vi "PCO_GetSegmentImageSettings.vi"(0 "ph":u64, 5 "wSegment":u16, 11 "error in (no error)":errorcluster {"code" format="%x"}) -> (1 "wRoiX1":u16, 2 "wRoiX0":u16, 3 "wBinHorz":u16, 4 "ph out":u64, 6 "ErrorMessage":i32 format="%x", 8 "wXRes":u16, 10 "wYRes":u16, 12 "wRoiY1":u16, 13 "wRoiY0":u16, 14 "wBinVert":u16, 15 "error out":errorcluster {"code" format="%x"})   [LabVIEW 2020, in "SDK.lvlib" / "ImageInformation.lvlib"]
doc: "<b>Description:</b>\nInformation about previously recorded images is queried from the camera. The returned parameters depend on the camera settings which have been active during the last recording to the dedicated segment.\n\n<b>Supported camera type:</b>\npco.dimax, pco.1200, pco1600, pco.2000, pco.4000\n\n<b>Descriptor dependency:</b>\ndwGeneralCapsDESC1: NO_RECORDER"
uses:
  ImageInformation.lvlib
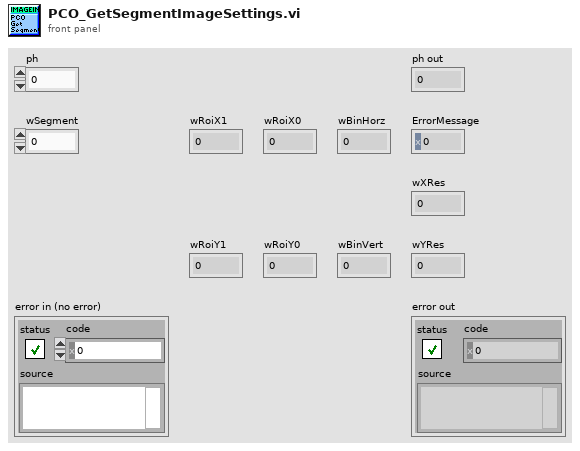
[diagram p1: front panel]
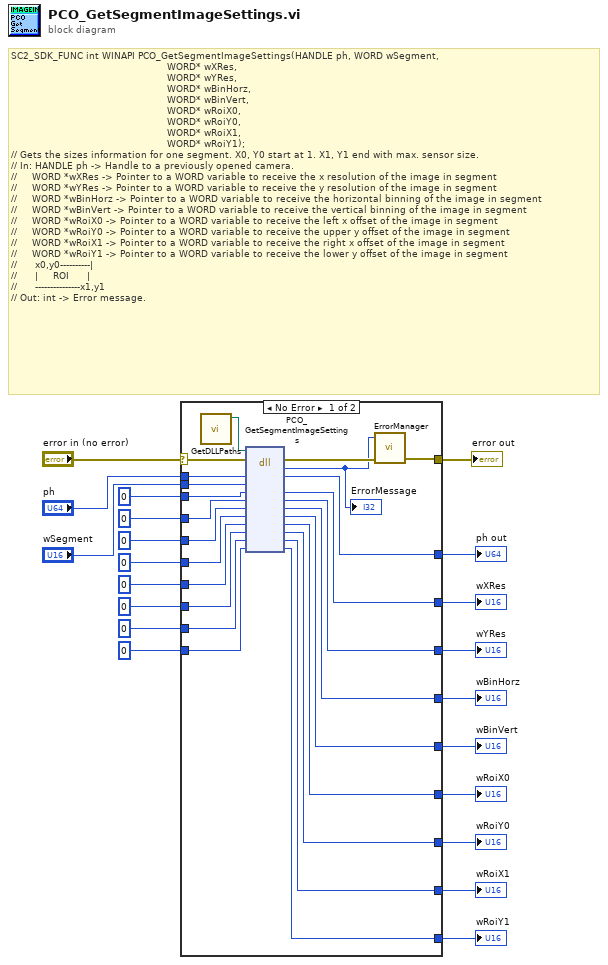
[diagram p0: block diagram]
diagram:
  # "SC2_SDK_FUNC int WINAPI PCO_GetSegmentImageSettings(HANDLE ph, WORD wSegment,\n                                                    WORD* wXRes,\n                                                    WORD* wYRes,\n                                                    WORD* wBinHorz,\n                                                    WORD* wBinVert,\n                                                    WORD* wRoiX0,\n                                                    WORD* wRoiY0,\n                                                    WORD* wRoiX1,\n                                                    WORD* wRoiY1);\n// Gets the sizes information for one segment. X0, Y0 start at 1. X1, Y1 end with max. sensor size.\n// In: HANDLE ph -> Handle to a previously opened camera.\n//     WORD *wXRes -> Pointer to a WORD variable to receive the x resolution of the image in segment\n//     WORD *wYRes -> Pointer to a WORD variable to receive the y resolution of the image in segment\n//     WORD *wBinHorz -> Pointer to a WORD variable to receive the horizontal binning of the image in segment\n//     WORD *wBinVert -> Pointer to a WORD variable to receive the vertical binning of the image in segment\n//     WORD *wRoiX0 -> Pointer to a WORD variable to receive the left x offset of the image in segment\n//     WORD *wRoiY0 -> Pointer to a WORD variable to receive the upper y offset of the image in segment\n//     WORD *wRoiX1 -> Pointer to a WORD variable to receive the right x offset of the image in segment\n//     WORD *wRoiY1 -> Pointer to a WORD variable to receive the lower y offset of the image in segment\n//      x0,y0----------|\n//      |     ROI      |\n//      ---------------x1,y1\n// Out: int -> Error message."
  n1 = case shown="No Error" "error in (no error)" {
    selector: "error in (no error)" -> [w23 w54]
    tunnel: "ph" -> [w45 w55]
    tunnel: [w44 w55] -> w20
    tunnel: "wSegment" -> [w43 _]
    tunnel: u16 0 ("wXRes") -> [w42 w53]
    tunnel: [w41 w53] -> w17
    tunnel: u16 0 ("wYRes") -> [w40 w52]
    tunnel: [w39 w52] -> w15
    tunnel: u16 0 ("wBinHorz") -> [w38 w51]
    tunnel: [w37 w51] -> w13
    tunnel: u16 0 ("wBinVert") -> [w36 w50]
    tunnel: [w35 w50] -> w11
    tunnel: u16 0 ("wRoiX0") -> [w34 w49]
    tunnel: [w33 w49] -> w9
    tunnel: u16 0 ("wRoiY0") -> [w32 w48]
    tunnel: [w31 w48] -> w7
    tunnel: u16 0 ("wRoiX1") -> [w30 w47]
    tunnel: [w29 w47] -> w5
    tunnel: u16 0 ("wRoiY1") -> [w28 w46]
    tunnel: [w27 w46] -> w3
    tunnel: [w25 w54] -> w2
    frame No Error {
      n2 = call "GetDLLPaths.vi"() -> ("SC2_Cam_Path"=w22:path)  [unwired: 9 in, 2 out]
      n3 = dll-call lib="?" fn="PCO_GetSegmentImageSettings"(path in=w22, error in=w23, "ph"=w45, "wSegment"=w43, "wXRes"=w42, "wYRes"=w40, "wBinHorz"=w38, "wBinVert"=w36, "wRoiX0"=w34, "wRoiY0"=w32, "wRoiX1"=w30, "wRoiY1"=w28) -> (error out=w26:errorcluster, "return type"=w24:i32, "ph"=w44:u64, "wXRes"=w41:u16, "wYRes"=w39:u16, "wBinHorz"=w37:u16, "wBinVert"=w35:u16, "wRoiX0"=w33:u16, "wRoiY0"=w31:u16, "wRoiX1"=w29:u16, "wRoiY1"=w27:u16)  [unwired: 2 in, 1 out]
      "ErrorMessage" <- w24
      n4 = call "ErrorManager.vi"("error in (no error)"=w26, "error code"=w24) -> ("error out"=w25:errorcluster)  [unwired: 3 in]
    }
    frame Error {
    }
  }
  "ph out" <- w20
  "wXRes" <- w17
  "wYRes" <- w15
  "wBinHorz" <- w13
  "wBinVert" <- w11
  "wRoiX0" <- w9
  "wRoiY0" <- w7
  "wRoiX1" <- w5
  "wRoiY1" <- w3
  "error out" <- w2
